vi "PwrSwpExample.vi"() -> ()   [LabVIEW 2018]
doc: "PNA-X Example."
uses:
  PNA-X.lvlib
panel:
  out "VISA Out":refnum<visa-resource-name>
  out "error out":errorcluster
  in  "error in":errorcluster
  in  "VNA Visa":refnum<visa-resource-name>
  # "1. Select Instrument Source from the \"VISA IN\" drop down.\n2. Run vi"
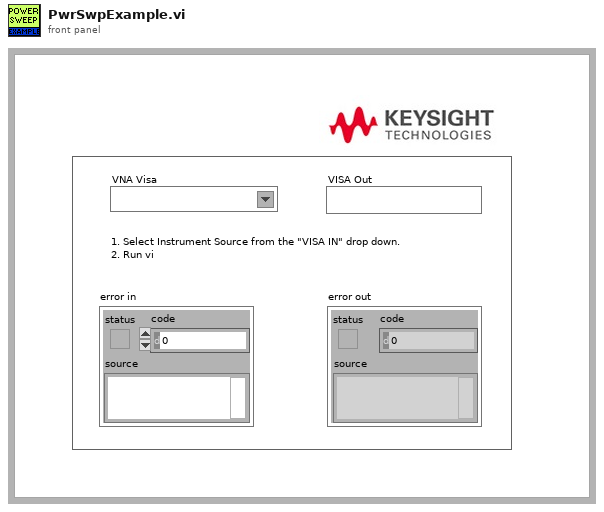
[diagram p1: front panel]
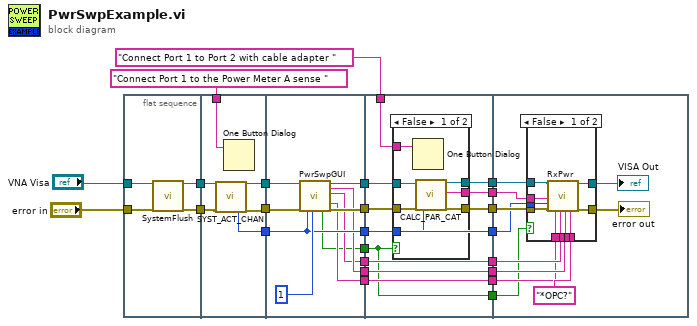
[diagram p0: block diagram]
diagram:
  n1 = flat-sequence {
    tunnel: "VNA Visa" -> [w28]
    tunnel: "error in" -> [w27]
    tunnel: [w26] -> w21
    tunnel: [w25] -> w20
    tunnel: "Connect Port 1 to the Power Meter A sense " -> [w34]
    tunnel: w21 -> [w33]
    tunnel: w20 -> [w32]
    tunnel: [w31] -> w19
    tunnel: [w30] -> w13
    tunnel: [w29] -> w4
    tunnel: w19 -> [w44]
    tunnel: [w42] -> w18
    tunnel: [w43] -> w17
    tunnel: w13 -> [w40]
    tunnel: [w40] -> w12
    tunnel: [w39] -> w10
    tunnel: [w38] -> w7
    tunnel: [w37] -> w5
    tunnel: w4 -> [w36]
    tunnel: [w35] -> w3
    tunnel: w18 -> [w51]
    tunnel: w17 -> [w52]
    tunnel: "Connect Port 1 to Port 2 with cable adapter " -> [w55]
    tunnel: [w54] -> w15
    tunnel: [w53] -> w14
    tunnel: w12 -> [w50]
    tunnel: [w50] -> w11
    tunnel: w10 -> [w49]
    tunnel: [w49] -> w9
    tunnel: [w48] -> w8
    tunnel: w7 -> [w48]
    tunnel: [w47] -> w6
    tunnel: w5 -> [w47]
    tunnel: w3 -> [w46]
    tunnel: [w46] -> w2
    tunnel: [w45] -> w1
    tunnel: w15 -> [w75]
    tunnel: w14 -> [w74]
    tunnel: w11 -> [w73]
    tunnel: w9 -> [w71]
    tunnel: w8 -> [w70]
    tunnel: w6 -> [w69]
    tunnel: w2 -> [w66]
    tunnel: w1 -> [w65]
    frame #0 {
      n2 = call "SystemFlush.vi"("VISA IN"=w28, "error in"=w27) -> ("VISA Out"=w26:refnum<visa-resource-name>, "error out"=w25:errorcluster)  [unwired: 16 in]
    }
    frame #1 {
      n3 = call "SYST_ACT_CHAN.vi"("VISA IN"=w33, "error in"=w32) -> ("Channel"=w30:i32, "VISA Out"=w29:refnum<visa-resource-name>, "error out"=w31:errorcluster)  [unwired: 15 in]
      n4 = One Button Dialog(message=w34) -> ()  [unwired: 1 in, 1 out]
    }
    frame #2 {
      n5 = call "PwrSwpGUI.vi"("VISA IN"=w36, "error in"=w44, "Channel"=w40, "Port"=1) -> ("Exit"=w35:bool, "VISA Out"=w42:refnum<visa-resource-name>, "Rx"=w39:string, "MethodOut"=w38:string, "MeasParameter"=w37:string, "error out"=w43:errorcluster)  [unwired: 9 in, 1 out]
    }
    frame #3 {
      n6 = case shown="False" w46 {
        tunnel: w55 -> [w62 _]
        tunnel: [w61 w64] -> w54
        tunnel: [w60 w63] -> w53
        tunnel: w52 -> [w59 w64]
        tunnel: w51 -> [w58 w63]
        tunnel: w50 -> [w57 _]
        tunnel: [w56 _] -> w45
        frame False {
          n7 = One Button Dialog(message=w62) -> ()  [unwired: 1 in, 1 out]
          n8 = call "CALC_PAR_CAT.vi"("VISA IN"=w58, "error in"=w59, "Channel"=w57) -> ("VISA Out"=w60:refnum<visa-resource-name>, "Data"=w56:string, "error out"=w61:errorcluster)  [unwired: 12 in, 2 out]
        }
        frame True {
        }
      }
    }
    frame #4 {
      n9 = case shown="False" w66 {
        tunnel: w75 -> [w85 w86]
        tunnel: w74 -> [w84 w87]
        tunnel: w73 -> [w83 _]
        tunnel: "*OPC?" ("Cmd") -> [w82 _]
        tunnel: w71 -> [w81 _]
        tunnel: w70 -> [w80 _]
        tunnel: w65 -> [w79 _]
        tunnel: w69 -> [w78 _]
        tunnel: [w77 w86] -> w68
        tunnel: [w76 w87] -> w67
        frame False {
          n10 = call "RxPwr.vi"("VISA IN"=w84, "Measurement"=w79, "Channel"=w83, "error in"=w85, "Measurement Parameter"=w78, "Method"=w80, "Receiver"=w81, "Cmd"=w82) -> ("VISA Out"=w76:refnum<visa-resource-name>, "error out"=w77:errorcluster)  [unwired: 10 in]
        }
        frame True {
        }
      }
      "error out" <- w68
      "VISA Out" <- w67
    }
  }
